vi "GenerateAttachablePosition_Bishop.vi"(1 "Black/White Turn (T/F)":bool, 2 "Board":i32[][](array[numeric])=[[-3, -5, -4, -1, -2, -4, -5, -3], [-6, -6, -6, -6, -6, -6, -6, -6], [0, 0, 0, 0, 0, 0, 0, 0], [0, 0, 0, 0, 0, 0, 0, 0], [0, 0, 0, 0, 0, 0, 0, 0], [0, 0, 0, 0, 0, 0, 0, 0], [6, 6, 6, 6, 6, 6, 6, 6], [3, 5, 4, 1, 2, 4, 5, 3]], 3 "pieceIndex":i32) -> (0 "AttachablePosition":bool[][](array[boolean]))   [LabVIEW 2014]
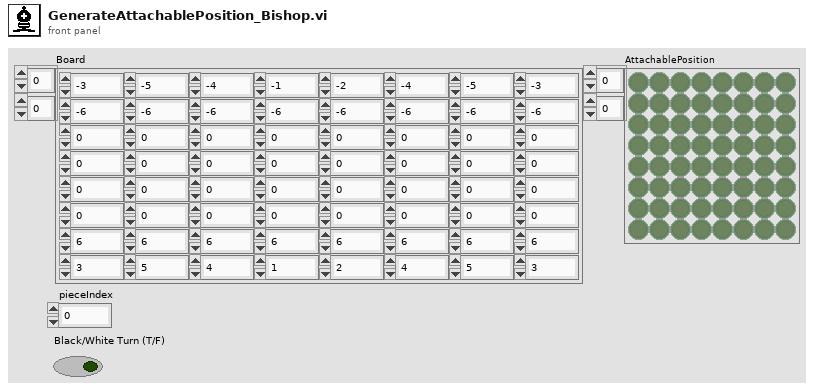
[diagram p1: front panel]
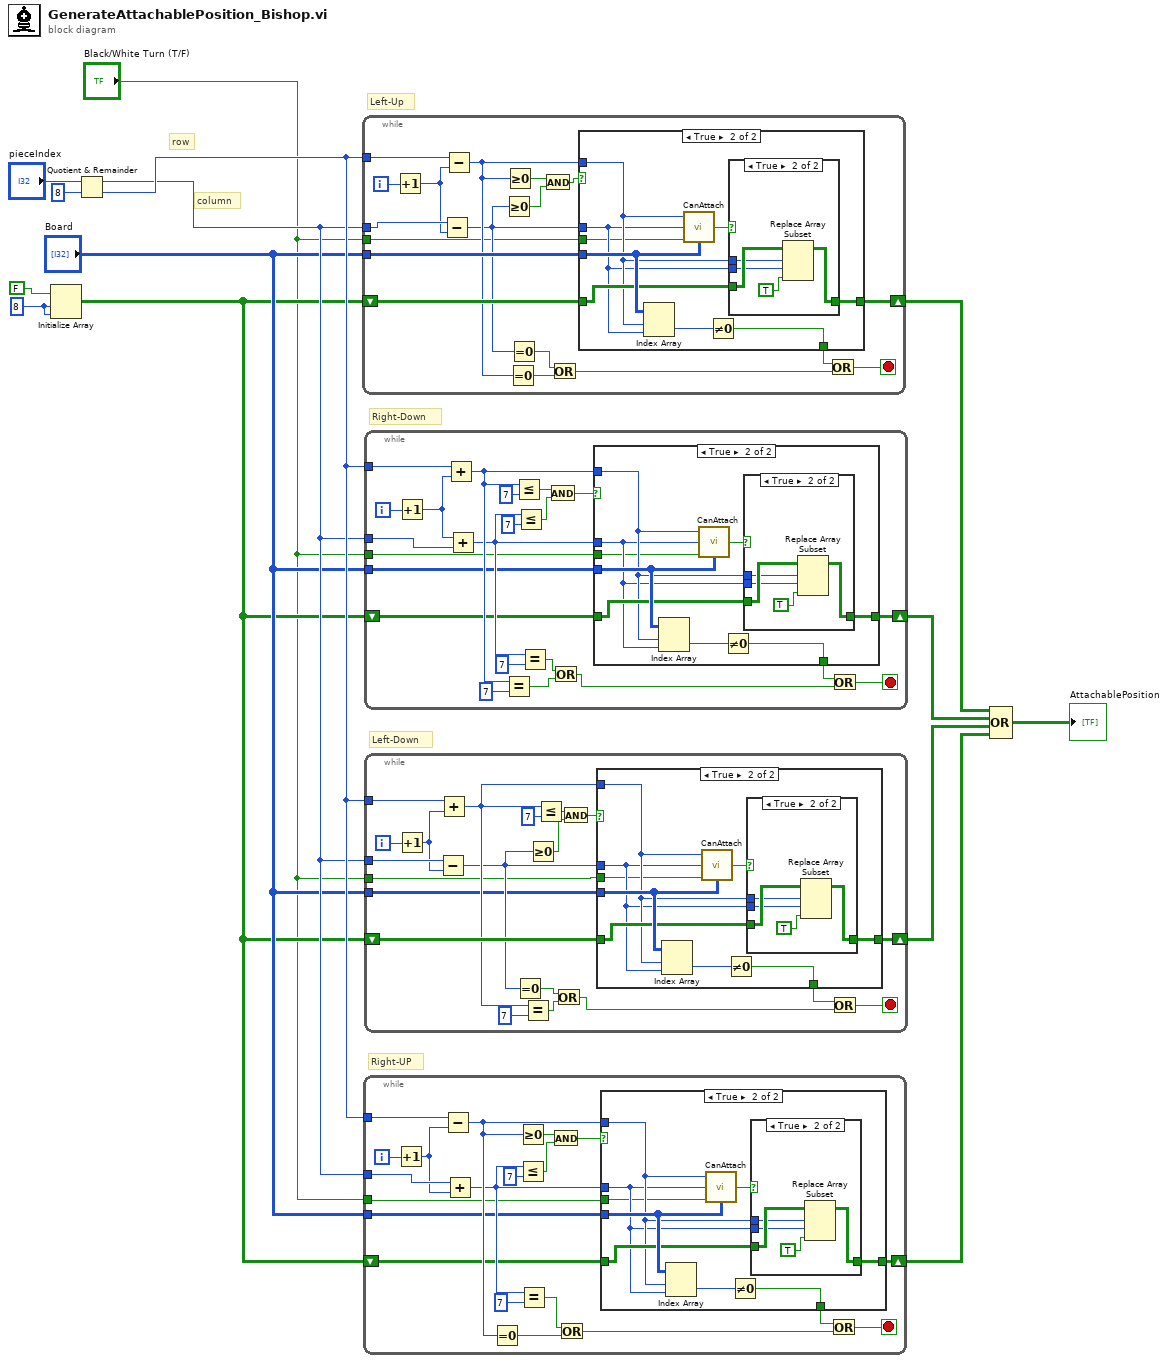
[diagram p0: block diagram]
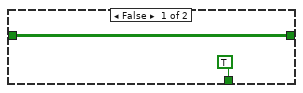
[diagram p2: hidden frame]
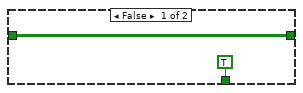
[diagram p4: hidden frame]
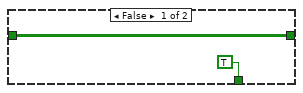
[diagram p6: hidden frame]
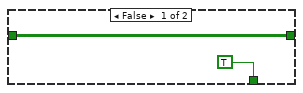
[diagram p8: hidden frame]
diagram:
  w12 = 8 ("dimension size")
  # "Right-UP"
  # "Left-Down"
  # "Right-Down"
  # "Left-Up"
  # "column"
  # "row"
  n1 = Initialize Array(FALSE, w12, w12) -> (w2:bool[][])
  n2 = Quotient & Remainder(x="pieceIndex", y=8) -> (x-y*floor(x/y)=w4:i32, floor(x/y)=w5:i32)
  n3 = while {
    tunnel: w5 -> [w30]
    tunnel: w4 -> [w23]
    tunnel: "Board" -> [w29]
    shift-right: [w27] -> w10
    shift-left: w2 -> [w28]
    tunnel: "Black/White Turn (T/F)" -> [w15]
    i -> [w32]
    stop <- w26 stop-if-true
    n4 = Increment(x=w32) -> (x+1=w22:i32)
    n5 = Subtract(x=w23, y=w22) -> (x-y=w16:i32)
    n6 = Subtract(x=w30, y=w22) -> (x-y=w24:i32)
    n7 = Greater Or Equal To 0?(x=w16) -> (x >= 0?=w20:bool)
    n8 = Greater Or Equal To 0?(x=w24) -> (x >= 0?=w31:bool)
    n9 = Equal To 0?(x=w24) -> (x = 0?=w18:bool)
    n10 = Equal To 0?(x=w16) -> (x = 0?=w17:bool)
    n11 = And(x=w31, y=w20) -> (x .and. y?=w21:bool)
    n12 = Or(x=w17, y=w18) -> (x .or. y?=w19:bool)
    n13 = case shown="True" w21 {
      tunnel: w24 -> [_ w37]
      tunnel: w16 -> [_ w36]
      tunnel: w29 -> [_ w41]
      tunnel: w28 -> [w34 w39]
      tunnel: [w34 w38] -> w27
      tunnel: [TRUE w42] -> w25
      tunnel: w15 -> [_ w35]
      frame False {
      }
      frame True {
        n14 = Index Array(array=w41, index (row)=w37, index (col)=w36) -> (element=w43:i32)
        n15 = call "CanAttach.vi"("Board"=w41, "Black/White Turn (T/F)"=w35, "Column"=w36, "Row"=w37) -> ("Boolean"=w40:bool)
        n16 = Not Equal To 0?(x=w43) -> (x != 0?=w42:bool)
        n17 = case shown="True" w40 {
          tunnel: w39 -> [w44 w48]
          tunnel: [w44 w47] -> w38
          tunnel: w37 -> [_ w46]
          tunnel: w36 -> [_ w45]
          frame False {
          }
          frame True {
            n18 = Replace Array Subset(array=w48, new element=TRUE ("new element/subarray"), index (row)=w46, index (col)=w45) -> (w47:bool[][])
          }
        }
      }
    }
    n19 = Or(x=w25, y=w19) -> (x .or. y?=w26:bool)
  }
  n20 = while {
    tunnel: w5 -> [w63]
    tunnel: w4 -> [w67]
    tunnel: "Board" -> [w54]
    shift-right: [w53] -> w6
    shift-left: w2 -> [w55]
    tunnel: "Black/White Turn (T/F)" -> [w52]
    i -> [w69]
    stop <- w68 stop-if-true
    n21 = Increment(x=w69) -> (x+1=w62:i32)
    n22 = Subtract(x=w63, y=w62) -> (x-y=w57:i32)
    n23 = Add(x=w67, y=w62) -> (x+y=w56:i32)
    n24 = Equal To 0?(x=w57) -> (x = 0?=w60:bool)
    n25 = Greater Or Equal To 0?(x=w57) -> (x >= 0?=w61:bool)
    n26 = Less Or Equal?(x=w56, y=7) -> (x <= y?=w64:bool)
    n27 = Equal?(x=w56, y=7) -> (x = y?=w58:bool)
    n28 = And(x=w61, y=w64) -> (x .and. y?=w50:bool)
    n29 = Or(x=w58, y=w60) -> (x .or. y?=w59:bool)
    n30 = case shown="True" w50 {
      tunnel: w57 -> [_ w74]
      tunnel: w56 -> [_ w73]
      tunnel: w54 -> [_ w78]
      tunnel: w55 -> [w71 w76]
      tunnel: [w71 w75] -> w53
      tunnel: [TRUE w79] -> w51
      tunnel: w52 -> [_ w72]
      frame False {
      }
      frame True {
        n31 = Index Array(array=w78, index (row)=w74, index (col)=w73) -> (element=w80:i32)
        n32 = call "CanAttach.vi"("Board"=w78, "Black/White Turn (T/F)"=w72, "Column"=w73, "Row"=w74) -> ("Boolean"=w77:bool)
        n33 = Not Equal To 0?(x=w80) -> (x != 0?=w79:bool)
        n34 = case shown="True" w77 {
          tunnel: w76 -> [w81 w85]
          tunnel: [w81 w84] -> w75
          tunnel: w74 -> [_ w83]
          tunnel: w73 -> [_ w82]
          frame False {
          }
          frame True {
            n35 = Replace Array Subset(array=w85, new element=TRUE ("new element/subarray"), index (row)=w83, index (col)=w82) -> (w84:bool[][])
          }
        }
      }
    }
    n36 = Or(x=w51, y=w59) -> (x .or. y?=w68:bool)
  }
  n37 = while {
    tunnel: w5 -> [w106]
    tunnel: w4 -> [w102]
    tunnel: "Board" -> [w91]
    shift-right: [w87] -> w9
    shift-left: w2 -> [w90]
    tunnel: "Black/White Turn (T/F)" -> [w92]
    i -> [w108]
    stop <- w105 stop-if-true
    n38 = Increment(x=w108) -> (x+1=w101:i32)
    n39 = Add(x=w106, y=w101) -> (x+y=w94:i32)
    n40 = Add(x=w101, y=w102) -> (x+y=w93:i32)
    n41 = Equal?(x=w94, y=7) -> (x = y?=w96:bool)
    n42 = Less Or Equal?(x=w94, y=7) -> (x <= y?=w107:bool)
    n43 = Less Or Equal?(x=w93, y=7) -> (x <= y?=w99:bool)
    n44 = Equal?(x=w93, y=7) -> (x = y?=w97:bool)
    n45 = And(x=w107, y=w99) -> (x .and. y?=w88:bool)
    n46 = Or(x=w97, y=w96) -> (x .or. y?=w95:bool)
    n47 = case shown="True" w88 {
      tunnel: w94 -> [_ w113]
      tunnel: w93 -> [_ w112]
      tunnel: w91 -> [_ w117]
      tunnel: w90 -> [w110 w115]
      tunnel: [w110 w114] -> w87
      tunnel: [TRUE w118] -> w89
      tunnel: w92 -> [_ w111]
      frame False {
      }
      frame True {
        n48 = Index Array(array=w117, index (row)=w113, index (col)=w112) -> (element=w119:i32)
        n49 = call "CanAttach.vi"("Board"=w117, "Black/White Turn (T/F)"=w111, "Column"=w112, "Row"=w113) -> ("Boolean"=w116:bool)
        n50 = Not Equal To 0?(x=w119) -> (x != 0?=w118:bool)
        n51 = case shown="True" w116 {
          tunnel: w115 -> [w120 w124]
          tunnel: [w120 w123] -> w114
          tunnel: w113 -> [_ w122]
          tunnel: w112 -> [_ w121]
          frame False {
          }
          frame True {
            n52 = Replace Array Subset(array=w124, new element=TRUE ("new element/subarray"), index (row)=w122, index (col)=w121) -> (w123:bool[][])
          }
        }
      }
    }
    n53 = Or(x=w89, y=w95) -> (x .or. y?=w105:bool)
  }
  n54 = while {
    tunnel: w5 -> [w139]
    tunnel: w4 -> [w143]
    tunnel: "Board" -> [w129]
    shift-right: [w133] -> w7
    shift-left: w2 -> [w132]
    tunnel: "Black/White Turn (T/F)" -> [w128]
    i -> [w145]
    stop <- w144 stop-if-true
    n55 = Increment(x=w145) -> (x+1=w138:i32)
    n56 = Subtract(x=w143, y=w138) -> (x-y=w130:i32)
    n57 = Add(x=w139, y=w138) -> (x+y=w131:i32)
    n58 = Equal To 0?(x=w130) -> (x = 0?=w134:bool)
    n59 = Equal?(x=w131, y=7) -> (x = y?=w135:bool)
    n60 = Greater Or Equal To 0?(x=w130) -> (x >= 0?=w142:bool)
    n61 = Less Or Equal?(x=w131, y=7) -> (x <= y?=w140:bool)
    n62 = Or(x=w134, y=w135) -> (x .or. y?=w136:bool)
    n63 = And(x=w140, y=w142) -> (x .and. y?=w126:bool)
    n64 = case shown="True" w126 {
      tunnel: w131 -> [_ w150]
      tunnel: w130 -> [_ w149]
      tunnel: w129 -> [_ w154]
      tunnel: w132 -> [w147 w152]
      tunnel: [w147 w151] -> w133
      tunnel: [TRUE w155] -> w127
      tunnel: w128 -> [_ w148]
      frame False {
      }
      frame True {
        n65 = Index Array(array=w154, index (row)=w150, index (col)=w149) -> (element=w156:i32)
        n66 = call "CanAttach.vi"("Board"=w154, "Black/White Turn (T/F)"=w148, "Column"=w149, "Row"=w150) -> ("Boolean"=w153:bool)
        n67 = Not Equal To 0?(x=w156) -> (x != 0?=w155:bool)
        n68 = case shown="True" w153 {
          tunnel: w152 -> [w157 w161]
          tunnel: [w157 w160] -> w151
          tunnel: w150 -> [_ w159]
          tunnel: w149 -> [_ w158]
          frame False {
          }
          frame True {
            n69 = Replace Array Subset(array=w161, new element=TRUE ("new element/subarray"), index (row)=w159, index (col)=w158) -> (w160:bool[][])
          }
        }
      }
    }
    n70 = Or(x=w127, y=w136) -> (x .or. y?=w144:bool)
  }
  n71 = Compound Arithmetic op=OR(w10, w9, w7, w6) -> (→"AttachablePosition":bool[][])
